vi "Set Force.vi"(8 "error in (no error)":errorcluster, 9 "Force Data":u8[](array[numeric]) format="%.0x", 10 "Force Active":bool, 11 "CIFChannels in":refnum<class "CIFChannels.lvclass">) -> (0 "error out":errorcluster, 3 "CIFChannels out":refnum<class "CIFChannels.lvclass">)   [LabVIEW 2021, in "CIFChannels.lvclass"]
uses:
  CIFChannels.lvclass
  CIFChannels.lvclass/CIFChannels.ctl
  Accessors/Write Forced.vi
  Accessors/Read Direction.vi
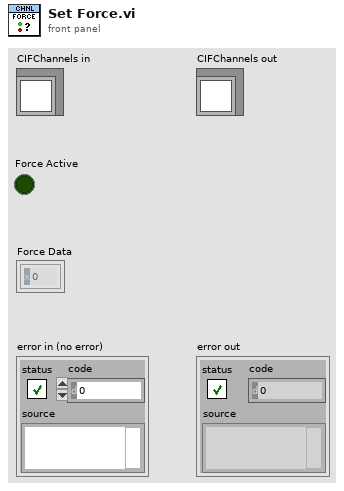
[diagram p1: front panel]
types:
  T1 = typedef "CIFChannels.lvclass/Direction.ctl" = enum16{"Publisher", "Subscriber"}
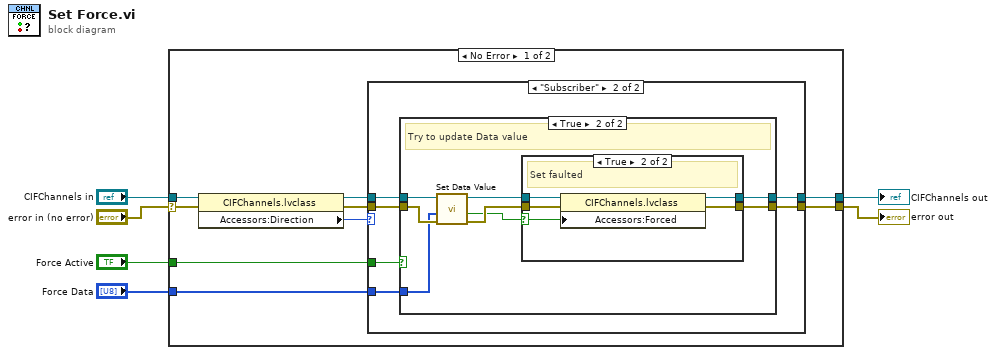
[diagram p0: block diagram]
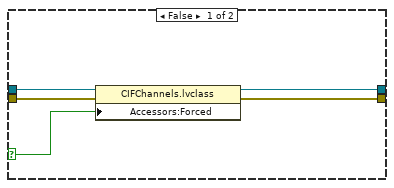
[diagram p3: hidden frame]
diagram:
  n1 = case shown="No Error" "error in (no error)" {
    selector: "error in (no error)" -> [w14 w45]
    tunnel: [w8 w45] -> w5
    tunnel: [w9 w44] -> w1
    tunnel: "CIFChannels in" -> [w15 w44]
    tunnel: "Force Active" -> [w10 _]
    tunnel: "Force Data" -> [w7 _]
    frame No Error {
      n2 = property class="CIFChannels.lvclass"(reference=w15, error in=w14) -> (reference out=w13:refnum<class "CIFChannels.lvclass">, error out=w11:errorcluster, "Accessors:Direction"=w12:T1)
      n3 = case shown="\"Subscriber\"" w12 {
        tunnel: w13 -> [w17 w22]
        tunnel: w11 -> [w16 w21]
        tunnel: w10 -> [_ w23]
        tunnel: [w17 w20] -> w9
        tunnel: [w16 w19] -> w8
        tunnel: w7 -> [_ w18]
        frame "Publisher" {
          # "Publisher can't be faulted.  Could add warning."
        }
        frame "Subscriber" {
          n4 = case shown="True" w23 {
            selector: w23 -> [w26 _]
            tunnel: w22 -> [w28 w36]
            tunnel: w21 -> [w27 w35]
            tunnel: [w25 w30] -> w20
            tunnel: [w24 w29] -> w19
            tunnel: w18 -> [_ w34]
            frame False {
              n5 = property class="CIFChannels.lvclass"(reference=w28, error in=w27, "Accessors:Forced"=w26) -> (reference out=w25:refnum<class "CIFChannels.lvclass">, error out=w24:errorcluster)
            }
            frame True {
              # "Try to update Data value"
              n6 = call-dynamic "Set Data Value.vi"("error in (no error)"=w35, "Flat Data"=w34, "CIFChannels in"=w36) -> ("error out"=w32:errorcluster, "Updated"=w31:bool, "CIFChannels out"=w33:refnum<class "CIFChannels.lvclass">)  [unwired: 6 in]
              n7 = case shown="True" w31 {
                selector: w31 -> [_ w41]
                tunnel: w33 -> [w38 w43]
                tunnel: w32 -> [w37 w42]
                tunnel: [w38 w40] -> w30
                tunnel: [w37 w39] -> w29
                frame False {
                  # "Update failed"
                }
                frame True {
                  # "Set faulted"
                  n8 = property class="CIFChannels.lvclass"(reference=w43, error in=w42, "Accessors:Forced"=w41) -> (reference out=w40:refnum<class "CIFChannels.lvclass">, error out=w39:errorcluster)
                }
              }
            }
          }
        }
      }
    }
    frame Error {
    }
  }
  "error out" <- w5
  "CIFChannels out" <- w1
